vi "NI9205_simpleUI_SaveData_OLD.vi"() -> ()   [LabVIEW 2020]
uses:
  TYPEDEF/NI9205_TD_Method.ctl
panel:
  in  "ClearData":bool
  in  "Save Now":bool
  out "Data size":i32
  in  "Nomefile_txt":string
  in  "file path":path
  out "Meter [kN]":dbl(knob) scale=0.0..100.0
  out "Waveform Graph 2":dbl[](graph)
  out "Spos mm":dbl
  out "V":dbl
  out "LC (kN)":dbl
  in  "q":dbl=2.15875
  in  "gain":dbl=-22.26172
  out "Waveform Graph":waveform(dbl)[](graph)
  in  "Stop":bool
  in  "Start":bool
  in  "Sample Rate":dbl=1000.0
  in  "Number of Samples":i32=100
  in  "Channels NI9205":tag="cDAQ2Mod2/ai6"
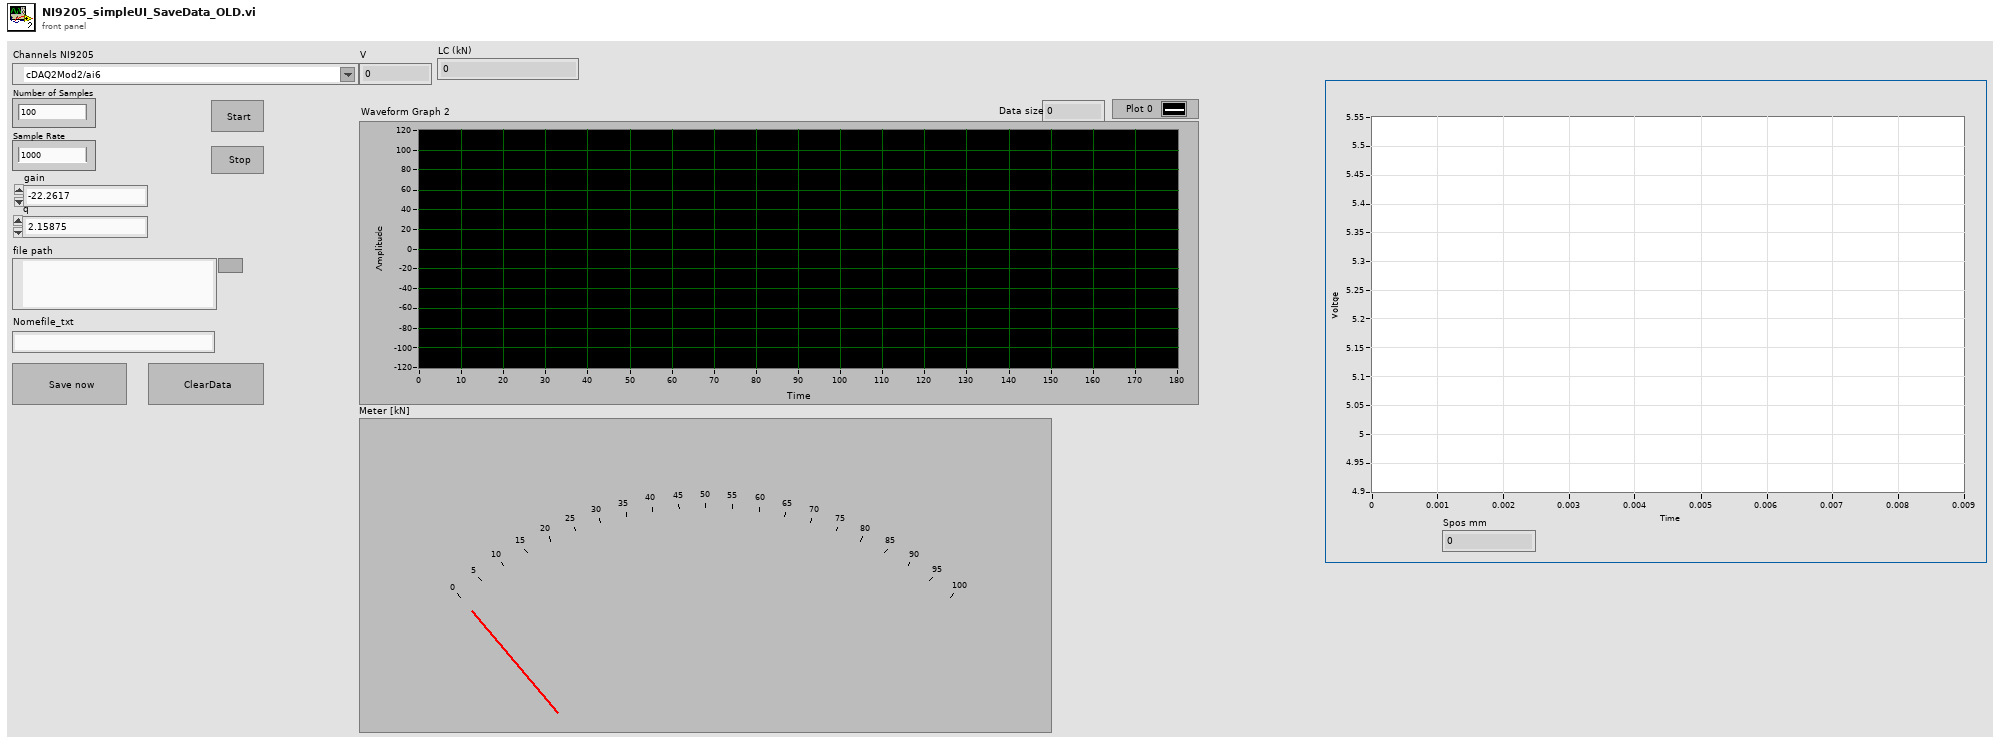
[diagram p1: front panel]
types:
  T1 = enum8{"Enabled", "Disabled", "Disabled and Grayed Out"}
  T2 = typedef "NI9205_TD_Method.ctl" = enum16{"NO_OP", "INIT", "SET", "GET", "CLOSE"}
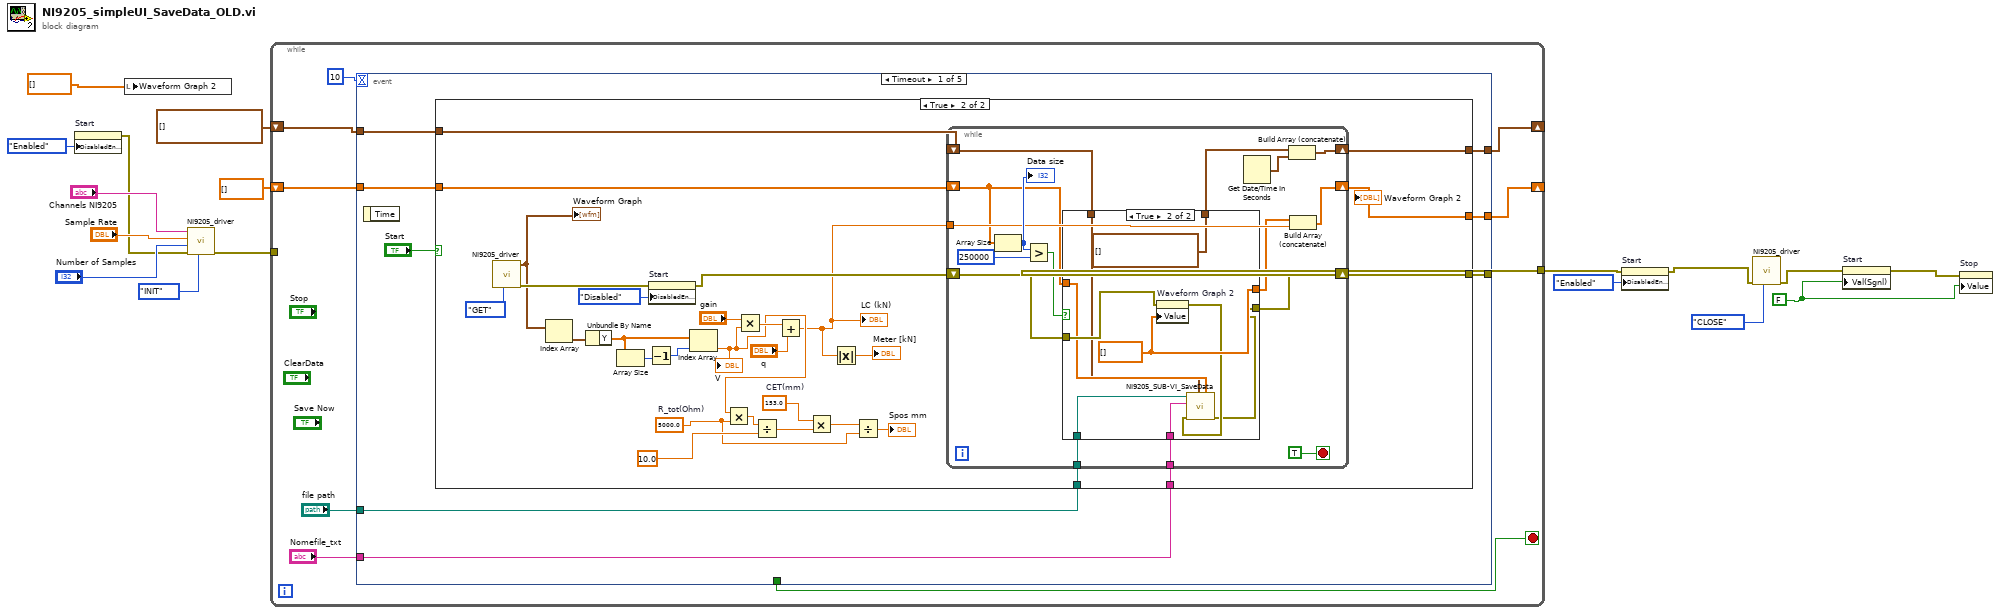
[diagram p0: block diagram]
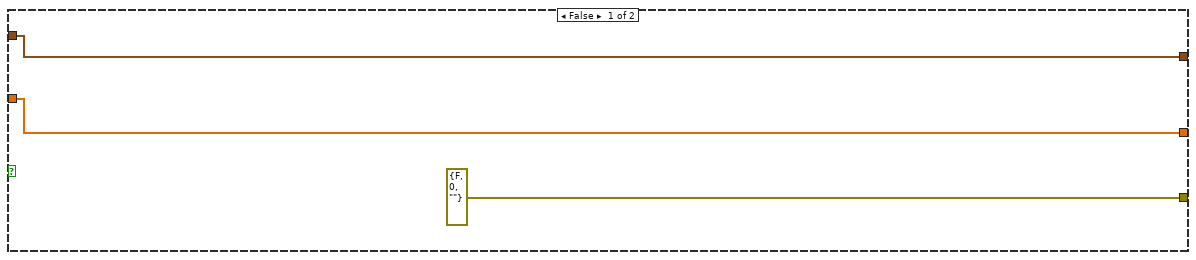
[diagram p2: hidden frame]
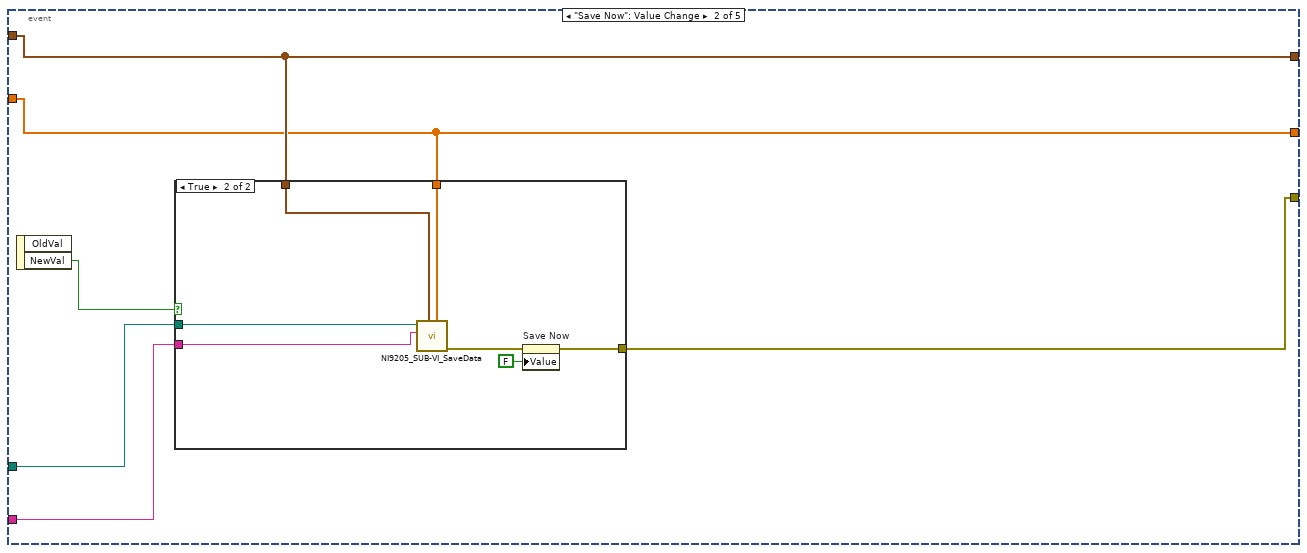
[diagram p4: hidden frame]
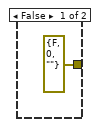
[diagram p5: hidden frame]
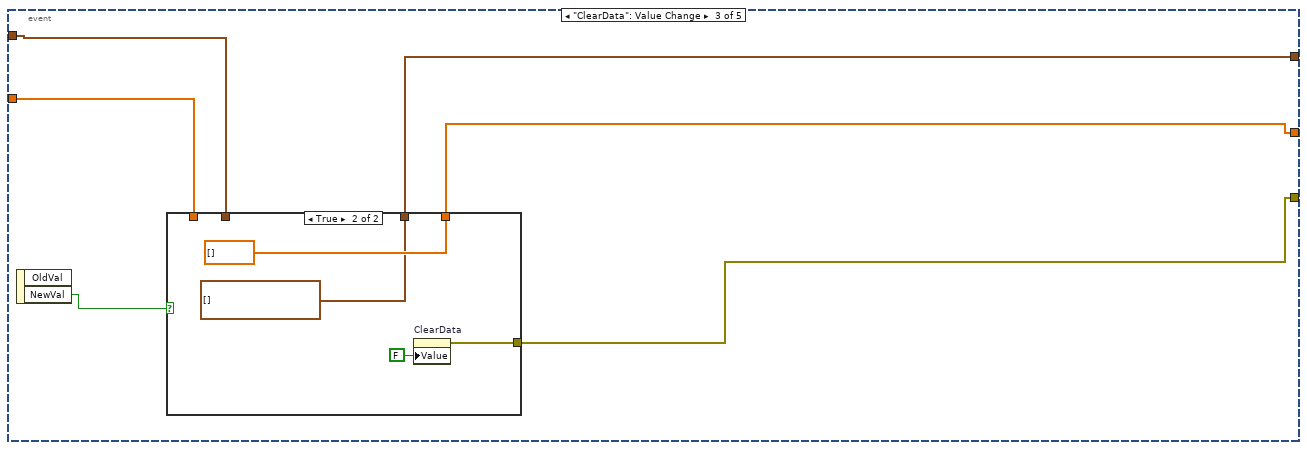
[diagram p6: hidden frame]
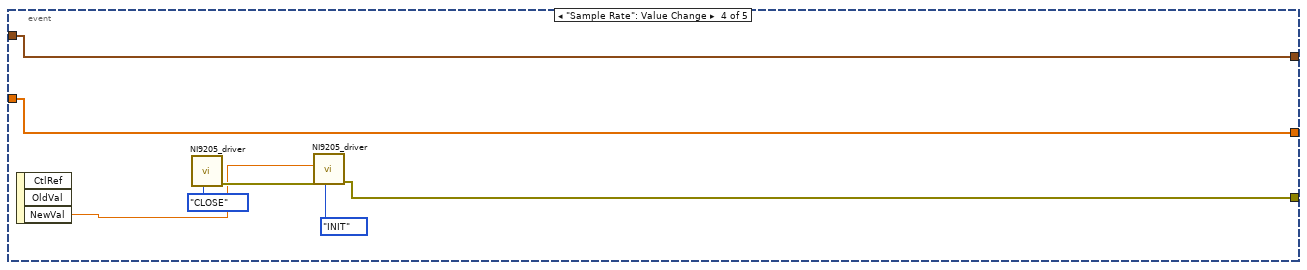
[diagram p8: hidden frame]
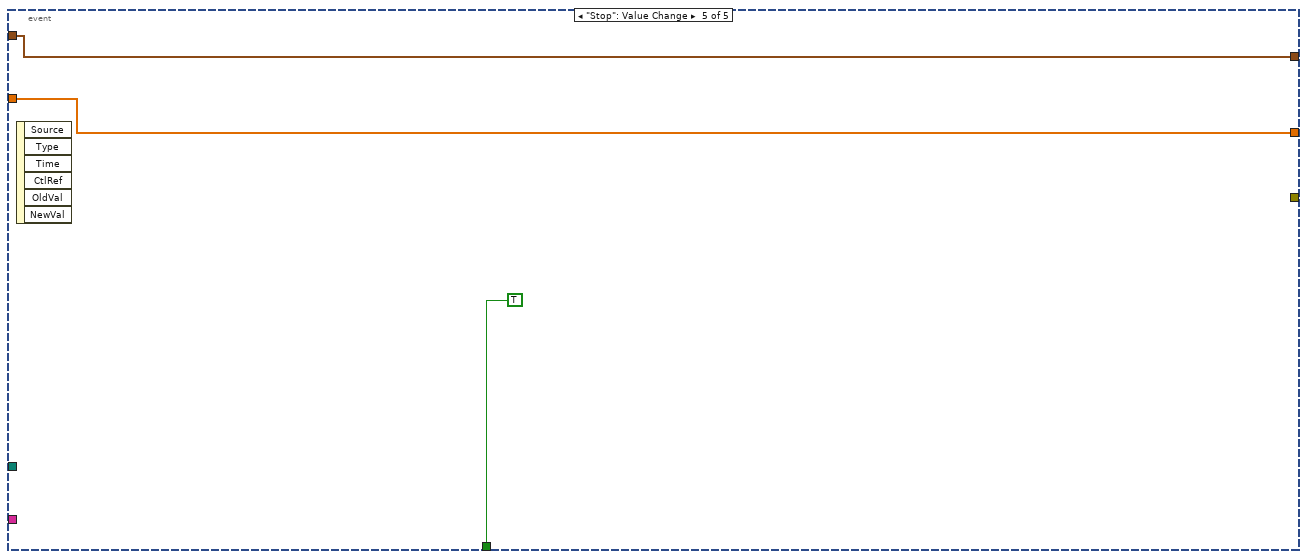
[diagram p9: hidden frame]
diagram:
  w6 = FALSE
  n1 = property on="Start" class="Bool (strict)"("DisabledEnum"=T1."Enabled" ("Disabled")) -> (error out=w3:errorcluster)  [unwired: 2 in, 1 out]
  n2 = local write "Waveform Graph 2"(dbl[] []) -> ()
  n3 = call "NI9205_driver.vi"("Method NI9205"=NI9205_TD_Method."INIT", "error in (no error)"=w3, "Number of Samples"="Number of Samples", "SampleRate"="Sample Rate", "Channels NI9205"="Channels NI9205") -> ("error out"=w13:errorcluster)  [unwired: 4 in, 2 out]
  n4 = while {
    tunnel: w13 -> [_]
    tunnel: [w26] -> w11
    shift-right: [w22] -> _
    shift-left: dbl[] [] -> [w23]
    shift-right: [w20] -> _
    shift-left: timestamp[] [] -> [w21]
    stop <- w25 stop-if-true
    n5 = event shown="[0] Timeout" {
      selector: _ -> [_ _ _ _ _]
      dyn-events: _ -> [_ _ _ _ _]
      timeout: 10 -> [_ _ _ _ _]
      tunnel: [w33 w95 w109 w123 _] -> w26
      tunnel: [_ _ _ _ TRUE] -> w25
      tunnel: w23 -> [w32 w98 w110 w122 w129]
      tunnel: [w31 w98 w113 w122 w129] -> w22
      tunnel: [w30 w99 w112 w121 w128] -> w20
      tunnel: w21 -> [w29 w99 w111 w121 w128]
      tunnel: "Nomefile_txt" -> [w28 w96 _ _ _]
      tunnel: "file path" -> [w27 w97 _ _ _]
      event Timeout {
        n6 = event-data() -> ()  [unwired: 1 in, 1 out]
        n7 = case shown="True" "Start" {
          tunnel: [errorcluster {"status"=FALSE, "code"=0, "source"=""} ("error out") w45] -> w33
          tunnel: w32 -> [w36 w43]
          tunnel: [w36 w42] -> w31
          tunnel: [w35 w41] -> w30
          tunnel: w29 -> [w35 w40]
          tunnel: w28 -> [_ w39]
          tunnel: w27 -> [_ w38]
          frame False {
          }
          frame True {
            w53 = 153.0  # CET(mm)
            w51 = 5000.0  # R_tot(Ohm)
            n8 = call "NI9205_driver.vi"("Method NI9205"=NI9205_TD_Method."GET") -> ("error out"=w65:errorcluster, "Waveform Graph"=w63:waveform(dbl)[])  [unwired: 8 in, 1 out]
            "Waveform Graph" <- w63
            n9 = Index Array(array=w63) -> (element=w62:waveform(dbl))  [unwired: 1 in]
            n10 = Unbundle By Name(w62) -> ("Y"=w61:dbl[])
            n11 = Array Size(array=w61) -> (size(s)=w60:i32)
            n12 = Decrement(x=w60) -> (x-1=w59:i32)
            n13 = property on="Start" class="Bool (strict)"(error in=w65, "DisabledEnum"=T1."Disabled" ("Disabled")) -> (error out=w46:errorcluster)  [unwired: 1 in, 1 out]
            n14 = Index Array(array=w61, index=w59) -> (element=w47:dbl)
            "V" <- w47
            n15 = Multiply(x=w47, y=w51) -> (x*y=w55:dbl)
            n16 = Multiply(x="gain", y=w47) -> (x*y=w57:dbl)
            n17 = Divide(x=w55, y=10.0 ("V_alim")) -> (x/y=w50:dbl)
            n18 = Add(x=w57, y="q") -> (x+y=w44:dbl)
            "LC (kN)" <- w44
            n19 = Multiply(x=w53, y=w50) -> (x*y=w52:dbl)
            n20 = Absolute Value(x=w44) -> (abs(x)=→"Meter [kN]":dbl)
            n21 = Divide(x=w52, y=w51) -> (x/y=→"Spos mm":dbl)
            n22 = while {
              shift-right: [w78] -> w45
              shift-left: w46 -> [w79]
              tunnel: w44 -> [w77]
              shift-right: [w76] -> w42
              shift-left: w43 -> [w73]
              shift-right: [w71] -> w41
              shift-left: w40 -> [w70]
              tunnel: w39 -> [w68]
              tunnel: w38 -> [w67]
              stop <- TRUE stop-if-true
              n23 = Array Size(array=w73) -> (size(s)=w82:i32)
              "Data size" <- w82
              n24 = Greater?(x=w82, y=250000) -> (0:w80:bool)
              n25 = case shown="True" w80 {
                tunnel: w79 -> [w85 w94]
                tunnel: [w85 w88] -> w78
                tunnel: w73 -> [w84 w92]
                tunnel: [w84 w93] -> w75
                tunnel: w70 -> [w83 w90]
                tunnel: [w83 timestamp[] []] -> w69
                tunnel: w68 -> [_ w87]
                tunnel: w67 -> [_ w86]
                frame False {
                }
                frame True {
                  w93 = dbl[] [] ("Waveform Graph 2")
                  n26 = property on="Waveform Graph 2" class="WFGraph (strict)"(error in=w94, "Value"=w93) -> (error out=w89:errorcluster)  [unwired: 1 in, 1 out]
                  n27 = call "NI9205_SUB-VI_SaveData.vi"("Arraych6"=w92, "Array Time"=w90, "error in (no error)"=w89, "Suffisso"=w87, "file path (use dialog)"=w86) -> ("error out"=w88:errorcluster)  [unwired: 5 in, 1 out]
                }
              }
              n28 = Get Date/Time In Seconds() -> (seconds since 1Jan1904=w72:timestamp)
              n29 = Build Array (concatenate)(w69, w72) -> (w71:timestamp[])
              n30 = Build Array (concatenate)(w75, w77) -> (w76:dbl[])
            }
            "Waveform Graph 2" <- w42
          }
        }
      }
      event "Save Now": Value Change {
        n31 = event-data() -> ("NewVal"=w100:bool)  [unwired: 1 in, 1 out]
        n32 = case shown="True" w100 {
          tunnel: w99 -> [_ w108]
          tunnel: w98 -> [_ w107]
          tunnel: w97 -> [_ w106]
          tunnel: w96 -> [_ w105]
          tunnel: [errorcluster {"status"=FALSE, "code"=0, "source"=""} ("error out") w102] -> w95
          frame False {
          }
          frame True {
            n33 = call "NI9205_SUB-VI_SaveData.vi"("Arraych6"=w107, "Array Time"=w108, "Suffisso"=w105, "file path (use dialog)"=w106) -> ("error out"=w103:errorcluster)  [unwired: 6 in, 1 out]
            n34 = property on="Save Now" class="Bool (strict)"(error in=w103, "Value"=FALSE ("Save Now")) -> (error out=w102:errorcluster)  [unwired: 1 in, 1 out]
          }
        }
      }
      event "ClearData": Value Change {
        n35 = event-data() -> ("NewVal"=w114:bool)  [unwired: 1 in, 1 out]
        n36 = case shown="True" w114 {
          tunnel: [w115 dbl[] []] -> w113
          tunnel: [w116 timestamp[] []] -> w112
          tunnel: w111 -> [w116 _]
          tunnel: w110 -> [w115 _]
          tunnel: [_ w117] -> w109
          frame False {
          }
          frame True {
            n37 = property on="ClearData" class="Bool (strict)"("Value"=FALSE ("ClearData")) -> (error out=w117:errorcluster)  [unwired: 2 in, 1 out]
          }
        }
      }
      event "Sample Rate": Value Change {
        n38 = event-data() -> ("NewVal"=w124:dbl)  [unwired: 1 in, 2 out]
        n39 = call "NI9205_driver.vi"("Method NI9205"=NI9205_TD_Method."CLOSE") -> ("error out"=w125:errorcluster)  [unwired: 8 in, 2 out]
        n40 = call "NI9205_driver.vi"("Method NI9205"=NI9205_TD_Method."INIT", "error in (no error)"=w125, "SampleRate"=w124) -> ("error out"=w123:errorcluster)  [unwired: 6 in, 2 out]
      }
      event "Stop": Value Change {
        n41 = event-data() -> ()  [unwired: 1 in, 6 out]
      }
    }
  }
  n42 = property on="Start" class="Bool (strict)"(error in=w11, "DisabledEnum"=T1."Enabled" ("Disabled")) -> (error out=w9:errorcluster)  [unwired: 1 in, 1 out]
  n43 = call "NI9205_driver.vi"("Method NI9205"=NI9205_TD_Method."CLOSE", "error in (no error)"=w9) -> ("error out"=w8:errorcluster)  [unwired: 7 in, 2 out]
  n44 = property on="Start" class="Bool (strict)"(error in=w8, "Val(Sgnl)"=w6) -> (error out=w7:errorcluster)  [unwired: 1 in, 1 out]
  n45 = property on="Stop" class="Bool (strict)"(error in=w7, "Value"=w6) -> ()  [unwired: 1 in, 2 out]
